vi "ProcessPlayerOperations.vi"(9 "WhoseTurn":u16, 10 "Players":T1[](array[typedef]), 11 "Game":T2) -> (1 "NewPlayers":T1[](array[typedef]), 3 "NewGame":T2)   [LabVIEW 2025]
uses:
  Controls/Game.ctl
  Controls/Player.ctl
panel:
  out "CurrentTile":u16
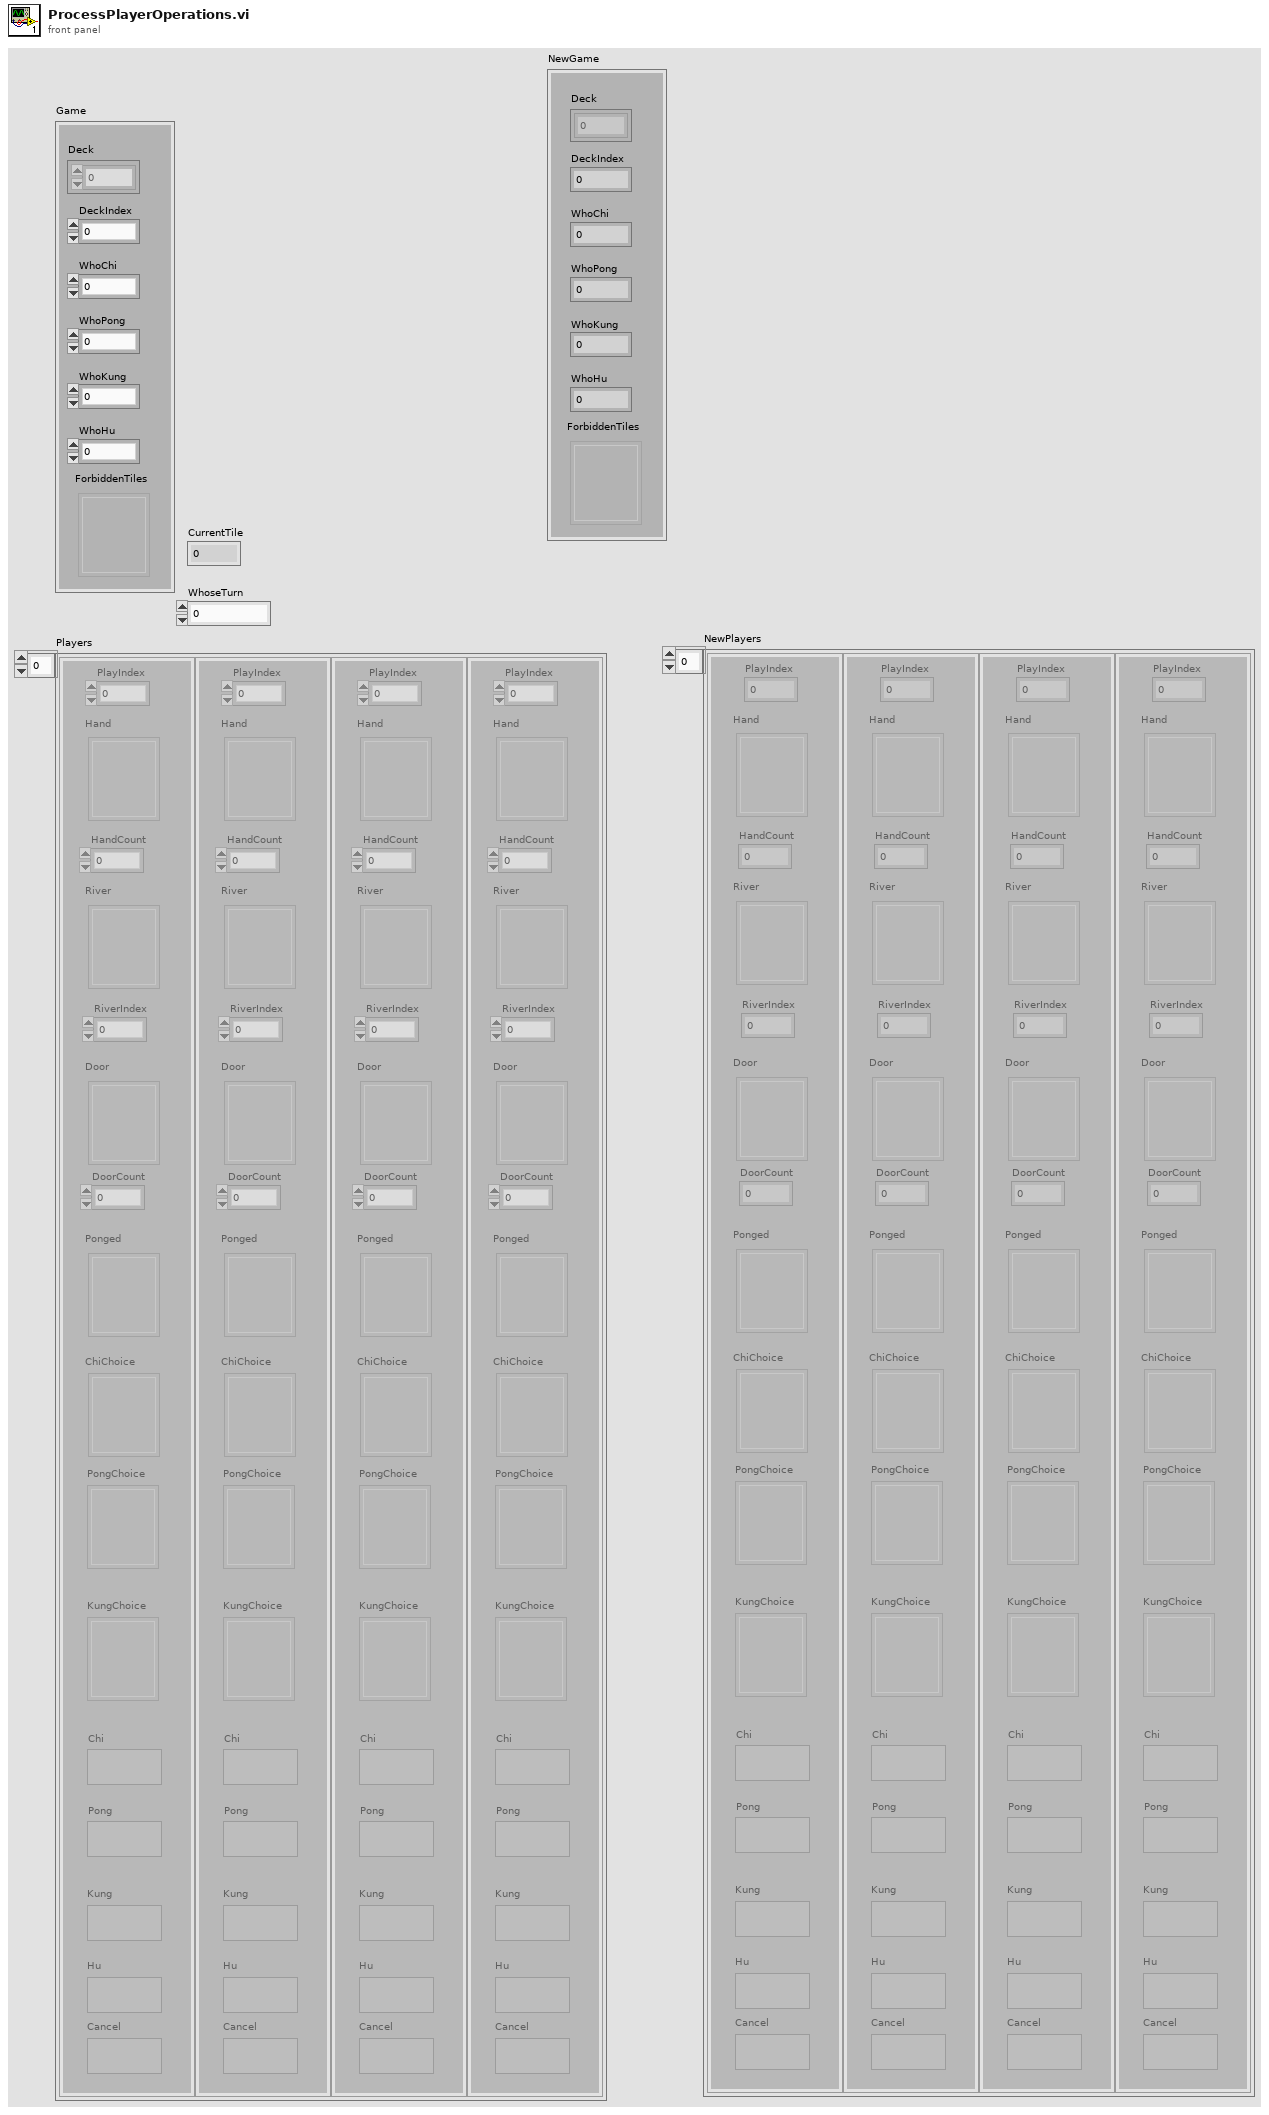
[diagram p1: front panel]
types:
  T1 = typedef "Player.ctl" = cluster{"PlayIndex":u16, "Hand":u16[], "HandCount":u16, "RiverIndex":u16, "Door":u16[], "DoorCount":u16, "Ponged":u16[], "ChiChoice":u16[][], "River":u16[][], "Chi":bool, "Pong":bool, "Kung":bool, "Hu":bool, "Cancel":bool, "PongChoice":u16, "KungChoice":u16}
  T2 = typedef "Game.ctl" = cluster{"DeckIndex":u16, "Deck":u16[], "WhoChi":u16, "WhoPong":u16, "WhoKung":u16, "WhoHu":u16, "ForbiddenTiles":u16[]}
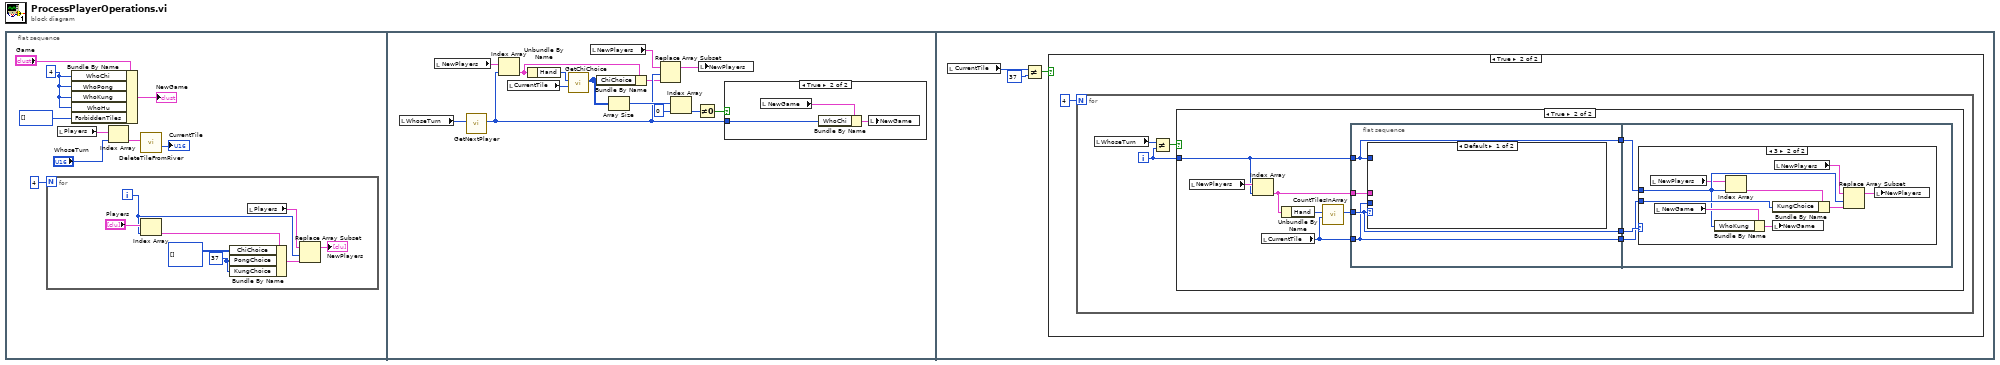
[diagram p0: block diagram]
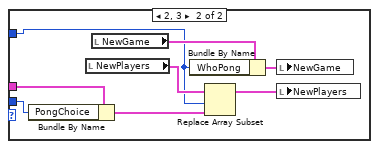
[diagram p5: hidden frame]
diagram:
  n1 = flat-sequence {
    frame #0 {
      w3 = 4
      n2 = for {
        N: 4 -> [_]
        i -> [w12]
        w14 = 37
        n3 = Index Array(array="Players", index=w12) -> (element=w16:T1)
        n4 = Bundle By Name(cluster=w16, "ChiChoice"=i32[][] [], "PongChoice"=w14, "KungChoice"=w14) -> (w13:T1)
        n5 = local read "Players"() -> (w11:T1[])
        n6 = Replace Array Subset(array=w11, new element=w13, index=w12) -> (→"NewPlayers":T1[])
      }
      n7 = local read "Players"() -> (w9:T1[])
      n8 = Bundle By Name(cluster="Game", "WhoChi"=w3, "WhoPong"=w3, "WhoKung"=w3, "WhoHu"=w3, "ForbiddenTiles"=i32[] []) -> (→"NewGame":T2)
      n9 = Index Array(array=w9, index="WhoseTurn") -> (element=w7:T1)
      n10 = call "DeleteTileFromRiver.vi"("Player"=w7) -> ("DeletedTile"=→"CurrentTile":u16)  [unwired: 9 in, 1 out]
    }
    frame #1 {
      n11 = local read "WhoseTurn"() -> (w29:u16)
      n12 = local read "NewPlayers"() -> (w30:T1[])
      n13 = call "GetNextPlayer.vi"("PlayerIndex"=w29) -> ("NewPlayerIndex"=w22:u16)  [unwired: 10 in]
      n14 = Index Array(array=w30, index=w22) -> (element=w24:T1)
      n15 = local read "CurrentTile"() -> (w18:u16)
      n16 = Unbundle By Name(w24) -> ("Hand"=w31:u16[])
      n17 = call "GetChiChoice.vi"("Tile"=w18, "Hand"=w31) -> ("ChiChoice"=w23:u16[][])  [unwired: 9 in]
      n18 = local read "NewPlayers"() -> (w20:T1[])
      n19 = Bundle By Name(cluster=w24, "ChiChoice"=w23) -> (w21:T1)
      n20 = Array Size(array=w23) -> (size(s)=w28:i32[])
      n21 = Replace Array Subset(array=w20, new element=w21, index=w22) -> (w19:T1[])
      n22 = Index Array(array=w28, index=0) -> (element=w26:i32)
      n23 = Not Equal To 0?(x=w26) -> (x != 0?=w25:bool)
      n24 = local write "NewPlayers"(w19) -> ()
      n25 = case shown="True" w25 {
        tunnel: w22 -> [_ w32]
        frame False {
        }
        frame True {
          n26 = local read "NewGame"() -> (w33:T2)
          n27 = Bundle By Name(cluster=w33, "WhoChi"=w32) -> (w34:T2)
          n28 = local write "NewGame"(w34) -> ()
        }
      }
    }
    frame #2 {
      n29 = local read "CurrentTile"() -> (w36:u16)
      n30 = Not Equal?(x=w36, y=37) -> (x != y?=w37:bool)
      n31 = case shown="True" w37 {
        frame False {
        }
        frame True {
          n32 = for {
            N: 4 -> [_]
            i -> [w40]
            n33 = local read "WhoseTurn"() -> (w41:u16)
            n34 = Not Equal?(x=w41, y=w40) -> (x != y?=w39:bool)
            n35 = case shown="True" w39 {
              tunnel: w40 -> [_ w47]
              frame False {
              }
              frame True {
                n36 = local read "NewPlayers"() -> (w50:T1[])
                n37 = Index Array(array=w50, index=w47) -> (element=w46:T1)
                n38 = local read "CurrentTile"() -> (w45:u16)
                n39 = Unbundle By Name(w46) -> ("Hand"=w49:u16[])
                n40 = call "CountTilesInArray.vi"("Tile"=w45, "Hand"=w49) -> ("Count"=w48:u16)  [unwired: 9 in]
                n41 = flat-sequence {
                  tunnel: w48 -> [w52]
                  tunnel: w47 -> [w54]
                  tunnel: w46 -> [w53]
                  tunnel: w45 -> [w51]
                  tunnel: [w54] -> w44
                  tunnel: [w52] -> w43
                  tunnel: [w51] -> w42
                  tunnel: w44 -> [w65]
                  tunnel: w43 -> [w64]
                  tunnel: w42 -> [w63]
                  frame #0 {
                    n42 = case shown="Default" w52 {
                      tunnel: w54 -> [_ w55]
                      tunnel: w53 -> [_ w57]
                      tunnel: w51 -> [_ w56]
                      frame Default {
                      }
                      frame 2, 3 {
                        n43 = Bundle By Name(cluster=w57, "PongChoice"=w56) -> (w60:T1)
                        n44 = local read "NewPlayers"() -> (w59:T1[])
                        n45 = local read "NewGame"() -> (w61:T2)
                        n46 = Bundle By Name(cluster=w61, "WhoPong"=w55) -> (w62:T2)
                        n47 = Replace Array Subset(array=w59, new element=w60, index=w55) -> (w58:T1[])
                        n48 = local write "NewGame"(w62) -> ()
                        n49 = local write "NewPlayers"(w58) -> ()
                      }
                    }
                  }
                  frame #1 {
                    n50 = case shown="3" w64 {
                      tunnel: w65 -> [_ w68]
                      tunnel: w63 -> [_ w69]
                      frame Default {
                      }
                      frame 3 {
                        n51 = local read "NewPlayers"() -> (w67:T1[])
                        n52 = local read "NewGame"() -> (w73:T2)
                        n53 = Bundle By Name(cluster=w73, "WhoKung"=w68) -> (w74:T2)
                        n54 = Index Array(array=w67, index=w68) -> (element=w66:T1)
                        n55 = Bundle By Name(cluster=w66, "KungChoice"=w69) -> (w72:T1)
                        n56 = local write "NewGame"(w74) -> ()
                        n57 = local read "NewPlayers"() -> (w71:T1[])
                        n58 = Replace Array Subset(array=w71, new element=w72, index=w68) -> (w70:T1[])
                        n59 = local write "NewPlayers"(w70) -> ()
                      }
                    }
                  }
                }
              }
            }
          }
        }
      }
    }
  }
